vi "rename_calls.vi"() -> ()   [LabVIEW 2014]
uses:
  <vilib>/Utility/traverseref.llb/TRef TravTarget.ctl
  <vilib>/Utility/traverseref.llb/VI Scripting - Traverse.lvlib
panel:
  out "processed VIs":string[](array[string])
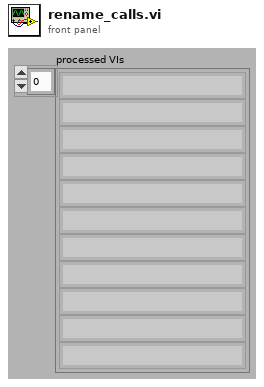
[diagram p1: front panel]
types:
  T1 = typedef "TRef TravTarget.ctl" = enum16{"FP", "BD", "Other"}
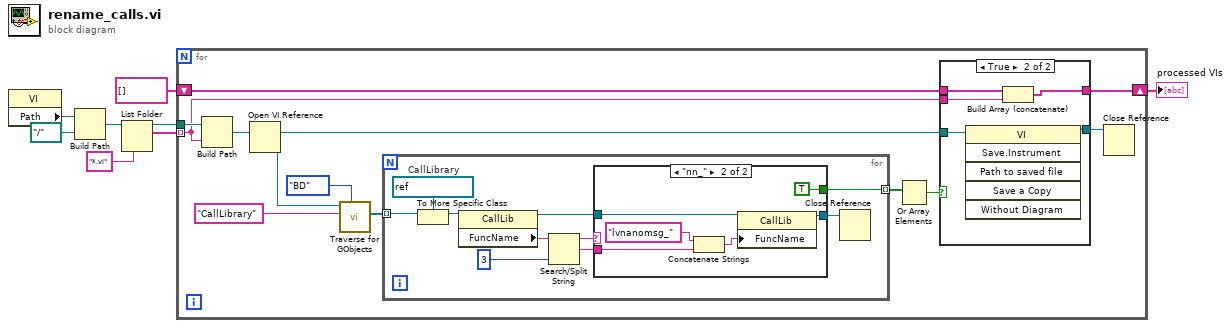
[diagram p0: block diagram]
diagram:
  n1 = property class="VI"() -> ("Path"=w1:path)  [unwired: 2 in, 2 out]
  n2 = Build Path(base path=w1, name or relative path=path "../.." ("Relative path (.)")) -> (appended path=w3:path)
  n3 = List Folder(path=w3, pattern="*.vi") -> (path out=w6:path, filenames=w7:string[])  [unwired: 2 in, 2 out]
  n4 = for {
    tunnel: w7 -> [w9] mode=indexing
    tunnel: w6 -> [w20]
    shift-right: [w10] -> w5
    shift-left: string[] [] -> [w11]
    n5 = Build Path(base path=w20, name or relative path=w9) -> (appended path=w19:path)
    n6 = Open VI Reference(vi path=w19) -> (vi reference=w14:refnum<vi>)  [unwired: 5 in, 1 out]
    n7 = call <vilib>:"Traverse for GObjects.vi"("Traverse Target"=TRef_TravTarget."BD", "Class Name"="CallLibrary", "VI Refnum"=w14) -> ("References"=w16:refnum<vi>[])  [unwired: 5 in, 3 out]
    n8 = for {
      tunnel: w16 -> [w37] mode=indexing
      tunnel: [w29] -> w15 mode=indexing
      w36 = refnum<vi> refnum  # CallLibrary
      n9 = To More Specific Class(target class=w36, reference=w37) -> (specific class reference=w35:refnum<vi>)  [unwired: 1 in, 1 out]
      n10 = property class="CallLib"(reference=w35) -> (reference out=w32:refnum<vi>, "FuncName"=w34:string)  [unwired: 1 in, 1 out]
      n11 = Search/Split String(string=w34, offset (0)=3 ("length (rest)")) -> (substring before match=w31:string, match + rest of string=w30:string)  [unwired: 1 in, 1 out]
      n12 = case shown="\"nn_\"" w31 {
        tunnel: w32 -> [w38 w44]
        tunnel: w30 -> [_ w43]
        tunnel: [_ TRUE] -> w29
        tunnel: [w38 w39] -> w28
        frame Default {
        }
        frame "nn_" {
          n13 = Concatenate Strings("lvnanomsg_" ("string"), w43) -> (w41:string)
          n14 = property class="CallLib"(reference=w44, "FuncName"=w41) -> (reference out=w39:refnum<vi>)  [unwired: 1 in, 1 out]
        }
      }
      n15 = Close Reference(reference=w28) -> ()  [unwired: 1 in, 1 out]
    }
    n16 = Or Array Elements(Boolean array=w15) -> (logical OR=w13:bool)
    n17 = case shown="True" w13 {
      tunnel: w14 -> [w22 w27]
      tunnel: [w22 w26] -> w12
      tunnel: w11 -> [w21 w25]
      tunnel: [w21 w24] -> w10
      tunnel: w9 -> [_ w23]
      frame False {
      }
      frame True {
        n18 = invoke class="VI" method="Save.Instrument"(reference=w27) -> (reference out=w26:refnum<vi>)  [unwired: 5 in, 5 out]
        n19 = Build Array (concatenate)(w25, w23) -> (w24:string[])
      }
    }
    n20 = Close Reference(reference=w12) -> ()  [unwired: 1 in, 1 out]
  }
  "processed VIs" <- w5
